vi "Local Client.vi"(6 "timeout (ms) [500]":i32=500, 8 "error in (no error)":errorcluster, 9 "params":variant, 10 "Command in":variant, 11 "Instrument in":refnum<class "Instrument.lvclass">) -> (0 "error out":errorcluster, 1 "Data out":variant, 2 "Command out":string, 3 "Instrument out":refnum<class "Instrument.lvclass">)   [LabVIEW 2019, in "Instrument.lvlib" / "Instrument.lvclass"]
doc: "Send a message to a local Instrument process. This VI is basically a wrapper for Instrument.sendMessageToProcess.vi with a mailbox to receive responses.\n\n<b>Command in</b> is a String. Conversion from Enum needs to be handled before calling this method (Use \"Enum to String.vi\")\n\n<b>Data in</b> is a Variant containing your data payload.\n\n<b>Data out</b> is a Variant."
uses:
  Instrument.lvclass
  c6c297fa-ccfe-4267-9780-fc415f7827cf.vi
  Instrument.sendMessageToProcess (variant).vi
  <vilib>/Utility/Data Type/Get Type Information.vi
  <vilib>/Utility/Data Type/Get Numeric Information.vi
  <userlib>/_OpenG.lib/lvdata/lvdata.llb/Unwrap VVariant__ogtk.vi
panel:
  # "Local Client.vi"
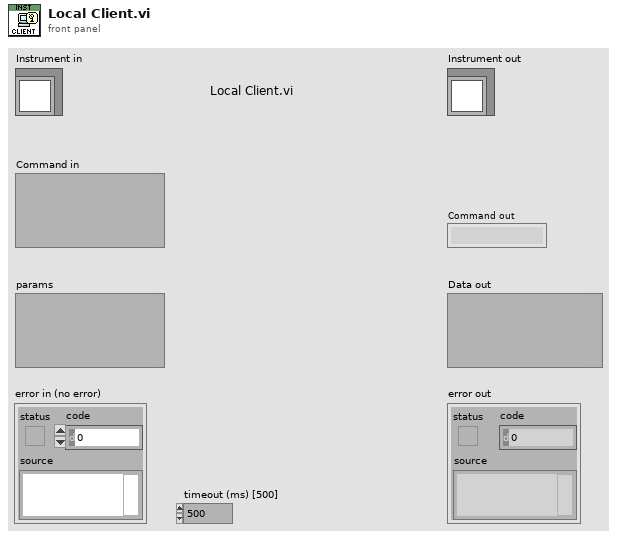
[diagram p1: front panel]
types:
  T1 = typedef "Instrument.lvlib/Instrument.lvclass/PublicEvents--Cluster.ctl" = cluster{"MessageFromProcess":refnum<user-event>}
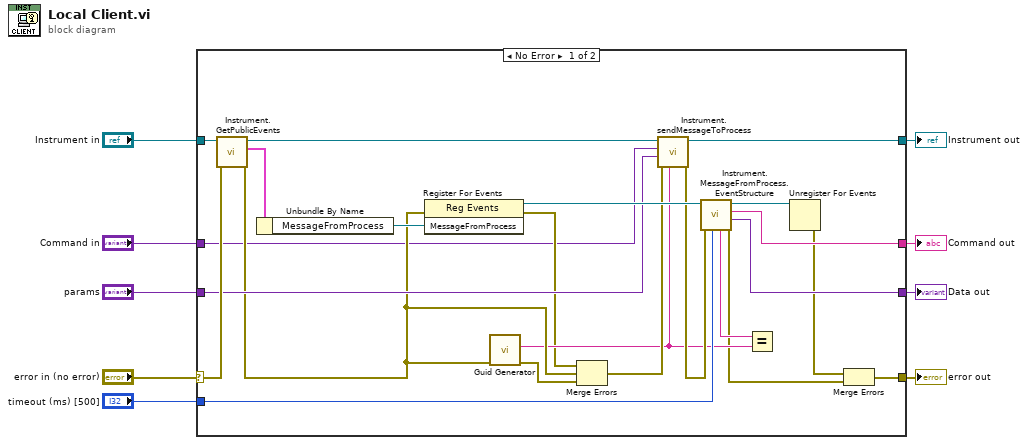
[diagram p0: block diagram]
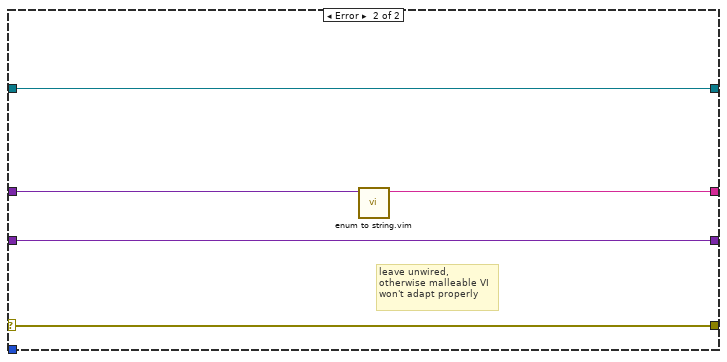
[diagram p2: hidden frame]
diagram:
  n1 = case shown="No Error" "error in (no error)" {
    selector: "error in (no error)" -> [w26 w37]
    tunnel: [w11 w37] -> w8
    tunnel: [w32 w36] -> w6
    tunnel: "Instrument in" -> [w28 w36]
    tunnel: "Command in" -> [w10 w33]
    tunnel: "params" -> [w19 w35]
    tunnel: "timeout (ms) [500]" -> [w21 _]
    tunnel: [w15 w34] -> w3
    tunnel: [w14 w35] -> w2
    frame No Error {
      n2 = call "Instrument.GetPublicEvents.vi"("error in (no error)"=w26, "Instrument"=w28) -> ("error out"=w18:errorcluster, "Instrument Public Events"=w31:T1, "Instrument out"=w27:refnum<class "Instrument.lvclass">)  [unwired: 7 in]
      n3 = Unbundle By Name(w31) -> ("MessageFromProcess"=w30:refnum<user-event>)
      n4 = register-events(error in=w18, w30) -> (reference out=w29:refnum<event-registration>, error out=w16:errorcluster)  [unwired: 1 in]
      n5 = call <vilib>:"Guid Generator.vi"("error in (no error)"=w18) -> ("error out"=w20:errorcluster, "GUID"=w17:string)  [unwired: 9 in]
      n6 = Merge Errors(w16, w18, w20) -> (w24:errorcluster)
      n7 = call-poly "Instrument.sendMessageToProcess.vi"("ID"=w17, "error in (no error)"=w24, "Data"=w19, "Command"=w10, "Instrument"=w27) -> ("error out"=w23:errorcluster, "Instrument out"=w32:refnum<class "Instrument.lvclass">)  [unwired: 5 in]
      n8 = call "Instrument.MessageFromProcess.EventStructure.vi"("timeout (ms) [500]"=w21, "error in (no error)"=w23, "Event Registration Refnum in"=w29) -> ("error out"=w13:errorcluster, "Data"=w14:variant, "Command"=w15:string, "Event Registration Refnum out"=w25:refnum<event-registration>, "ID"=w22:string)  [unwired: 4 in]
      n9 = Equal?(x=w22, y=w17) -> ()  [unwired: 1 out]
      n10 = Unregister For Events(event registration refnum=w25) -> (error out=w12:errorcluster)  [unwired: 1 in]
      n11 = Merge Errors(w12, w13) -> (w11:errorcluster)
    }
    frame Error {
      # "leave unwired,\notherwise malleable VI\nwon't adapt properly"
      n12 = call "enum to string.vim"("enum in"=w33) -> ("string out"=w34:string)  [unwired: 9 in, 1 out]
    }
  }
  "error out" <- w8
  "Instrument out" <- w6
  "Command out" <- w3
  "Data out" <- w2
